vi "SetError.vi"(6 "error in":errorcluster, 7 "Zusatzinfo zum Fehler":string, 8 "error code":i32=9000 min=5000 max=9999, 9 "Error?":bool) -> (0 "error out":errorcluster)   [LabVIEW 2021]
doc: "Dieses VI setzt einen Error (=error code) ab. Die Errornummer muss von 5000 ....? liegen (5000...9999 sind reserviert benutzerspeifische Fehler). Dem String Control können Zusatzinformationen direkt aus dem Source Code (z.B. für Debugging) übergeben werden, welche NICHT im error.txt aufgeführt sind.\n\nÜber den Boolean Eingang: Error? wird der Error aktiviert.\nDer Fehler wird nur gesetzt, wenn ErrorIN nicht gesetzt ist. Damit werden Folgefehler vermieden. Hingegen werden anliegende Warnungen durch einen Fehler überschrieben.s\n\nR. Egli / Zühlke Engineering AG\n07. Februar 03"
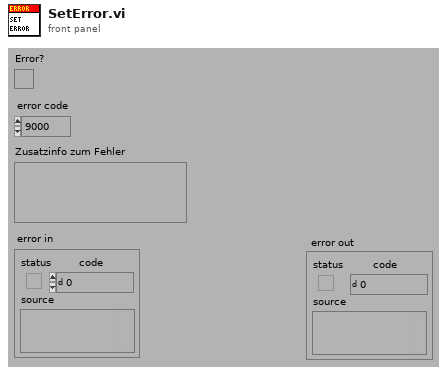
[diagram p1: front panel]
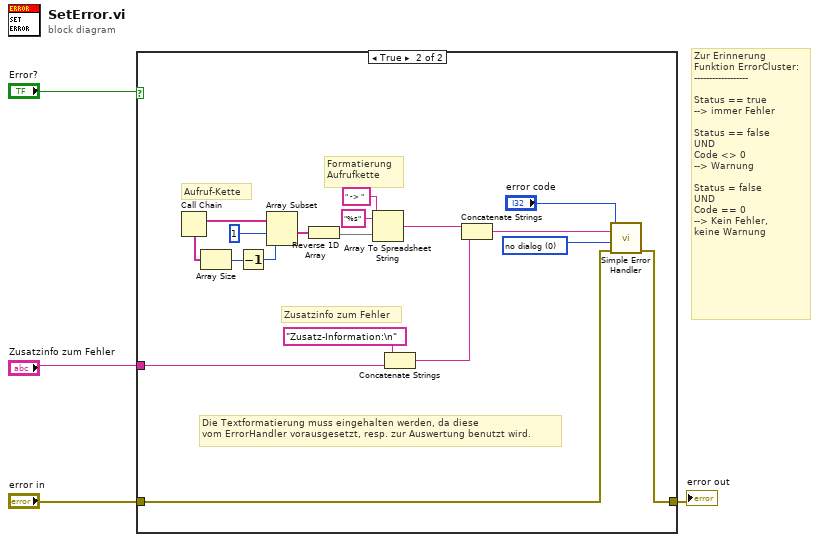
[diagram p0: block diagram]
diagram:
  # "Zur Erinnerung\nFunktion ErrorCluster:\n------------------\n\nStatus == true\n--> immer Fehler\n\nStatus == false\nUND \nCode <> 0 \n--> Warnung\n\nStatus = false\nUND \nCode == 0\n--> Kein Fehler,\nkeine Warnung"
  n1 = case shown="True" "Error?" {
    tunnel: [w5 w22] -> w4
    tunnel: "error in" -> [w5 w13]
    tunnel: "Zusatzinfo zum Fehler" -> [_ w8]
    frame False {
      # "ErrorCode = 0,\nes gibt nichts zu tun"
    }
    frame True {
      w6 = 0 items=["no dialog", "OK message", "continue or stop message"] ("type of dialog (OK msg:1)")
      # "Formatierung \nAufrufkette"
      # "Die Textformatierung muss eingehalten werden, da diese\nvom ErrorHandler vorausgesetzt, resp. zur Auswertung benutzt wird."
      # "Zusatzinfo zum Fehler"
      # "Aufruf-Kette"
      n2 = Call Chain() -> (call chain=w21:string[])
      n3 = Array Size(array=w21) -> (size(s)=w18:i32)
      n4 = Decrement(x=w18) -> (x-1=w19:i32)
      n5 = Array Subset(array=w21, index=1, length=w19) -> (w15:string[])
      n6 = Reverse 1D Array(array=w15) -> (reversed array=w16:string[])
      n7 = Array To Spreadsheet String(delimiter (Tab)=" -> ", array=w16, 3:"%s" ("format string")) -> (spreadsheet string=w12:string)
      n8 = Concatenate Strings("Zusatz-Information:\n", w8) -> (w11:string)
      n9 = Concatenate Strings(w12, w11) -> (w9:string)
      n10 = call <vilib>:"Simple Error Handler.vi"("error code (no error:0)"="error code", "error source (\" \")"=w9, "type of dialog (OK msg:1)"=w6, "error in (no error)"=w13) -> ("error out"=w22:errorcluster)  [unwired: 1 in, 4 out]
    }
  }
  "error out" <- w4
